vi "WLAN - niVST - RFSG - HWSetting.vi"(7 "numPackets":i32=100, 8 "Address String":string="00:90:4C:C5:12:38", 9 "ScriptName<index>":string="WLANRxTesting", 10 "Rx Measurements Settings":T2={"Standard"=4, "Channel Bandwidth (Hz)"=40000000.0, "Idle Interval (s)"=0.0001, "MCS Index"=0, "80211n PLCP Frame Format"=0, "Payload Data Length (bytes)"=1024, "OFDM Data Rate (Mbps)"=0, "DSSS Data Rate (Mbps)"=0, "# Packets"=0, "Carrier Frequency(Hz)"=5180000000.0, "Sweep Settings"={"Stop Power Level(dBm)"=-25.0, "Start Power Level(dBm)"=-25.0, "Step Size"=1.0}, "#N_SS"=0} {"DSSS Data Rate (Mbps)" items=["1", "2", "5.5 CCK", "5.5 PBCC", "11 CCK", "11 PBCC", "22", "33"]; "OFDM Data Rate (Mbps)" items=["6", "9", "12", "18", "24", "36", "48", "54"]; "80211n PLCP Frame Format" items=["Mixed Format", "Greenfield Format"]; "Standard" items=["80211A/G/J/P OFDM", "80211B/G DSSS", "80211G DSSSOFDM", "80211N MIMOOFDM", "80211AC MIMOOFDM"]}, 11 "instrument handle":refnum<k15>="pxi1slot2") -> (0 "PER Sweep Settings":T1, 1 "actual headroom (dB)":dbl, 2 "IQRate":dbl, 3 "RFSG handle out":refnum<k15>, 5 "error out":errorcluster)   [LabVIEW 2012]
uses:
  TV/RW/Includes/WLAN - TV - OPPO - RW - INC - TV_Rx_Measurements.ctl
  TV/RW/Includes/WLAN - TV - RW - INC - Rx_PER_Sweep_Settings.ctl
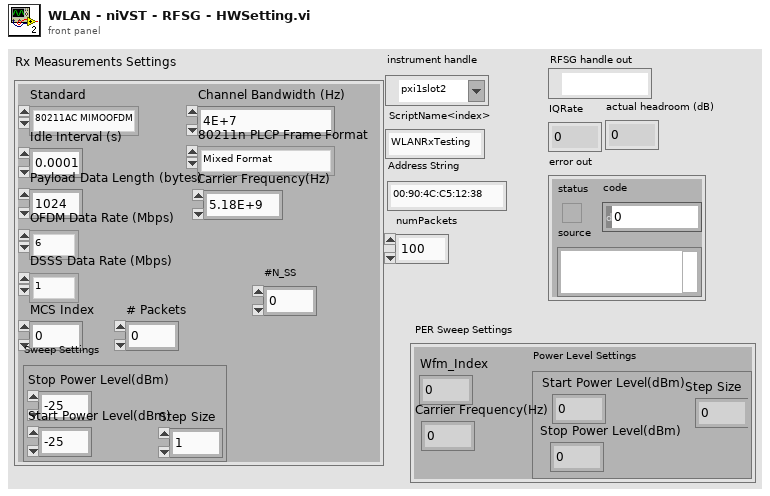
[diagram p1: front panel]
types:
  T1 = typedef "WLAN - TV - RW - INC - Rx_PER_Sweep_Settings.ctl" = cluster{"Wfm_Index":i32, "Power Level Settings":cluster{"Stop Power Level(dBm)":dbl, "Start Power Level(dBm)":dbl, "Step Size":dbl}, "Carrier Frequency(Hz)":dbl}
  T2 = typedef "WLAN - TV - OPPO - RW - INC - TV_Rx_Measurements.ctl" = cluster{"Standard":i32, "Channel Bandwidth (Hz)":dbl, "Idle Interval (s)":dbl, "MCS Index":i32, "80211n PLCP Frame Format":i32, "Payload Data Length (bytes)":i32, "OFDM Data Rate (Mbps)":i32, "DSSS Data Rate (Mbps)":i32, "# Packets":i32, "Carrier Frequency(Hz)":dbl, "Sweep Settings":cluster{"Stop Power Level(dBm)":dbl, "Start Power Level(dBm)":dbl, "Step Size":dbl}, "#N_SS":i32}
  T3 = typedef "WLAN - TV - RW - INC - Rx_PER_Wfm_Settings.ctl" = cluster{"Standard":i32, "Channel Bandwidth (Hz)":dbl, "Idle Interval (s)":dbl, "MCS Index":i32, "80211n PLCP Frame Format":i32, "Payload Data Length (bytes)":i32, "OFDM Data Rate (Mbps)":i32, "DSSS Data Rate (Mbps)":i32, "Wfm_Index":i32, "#N_SS":i32}
  T4 = typedef "WLAN - TV - RW - INC - RxTestParameters.ctl" = cluster{"wfm Size in msec":i32, "actual headroom (dB)":dbl, "Size in Samples":i32[], "40M?":bool, "Standard ":i32, "wfm size sec (dbl)":dbl, "dt":dbl, "Channel Bandwidth (Hz)":dbl, "Payload Data Length (bytes)":i32, "80211n PLCP Frame Format":i32, "DSSS Data Rate (Mbps)":i32, "OFDM Data Rate (Mbps)":i32, "MCS Index":i32, "Fc(Hz)":dbl, "#Packets":i32, "#N_SS":i32}
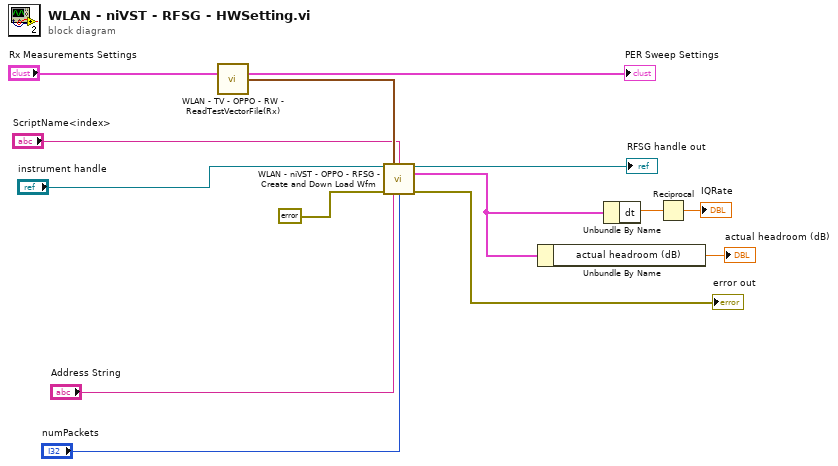
[diagram p0: block diagram]
diagram:
  n1 = call "WLAN - TV - OPPO - RW - ReadTestVectorFile(Rx).vi"("Rx Measurements Settings"="Rx Measurements Settings") -> ("PER Sweep Settings"=→"PER Sweep Settings":T1, "Waveform Generation Settings"=w12:T3)  [unwired: 13 in]
  n2 = call "WLAN - niVST - OPPO - RFSG - Create and Down Load Wfm.vi"("instrument handle"="instrument handle", "Rx Measurements Settings"=w12, "ScriptName<index>"="ScriptName<index>", "error in"=errorcluster {"status"=FALSE, "code"=0, "source"=""}, "Address String"="Address String", "numPackets"="numPackets") -> ("instrument handle"=→"RFSG handle out":refnum<k15>, "Rx_Test Parameters"=w5:T4, "error out"=→"error out":errorcluster)  [unwired: 7 in]
  n3 = Unbundle By Name(w5) -> ("actual headroom (dB)"=→"actual headroom (dB)":dbl)
  n4 = Unbundle By Name(w5) -> ("dt"=w7:dbl)
  n5 = Reciprocal(x=w7) -> (1/x=→"IQRate":dbl)
